vi "FGV_viertel_kreis_1Q.vi"(8 "error in (no error)":errorcluster, 9 "Sektor":T1, 11 "mode":T2) -> (0 "error out":errorcluster, 1 "size":i32, 3 "Q":dbl[][](array[numeric]) format="%_2g")   [LabVIEW 2019]
uses:
  mode_Q.ctl
  Quadrant.ctl
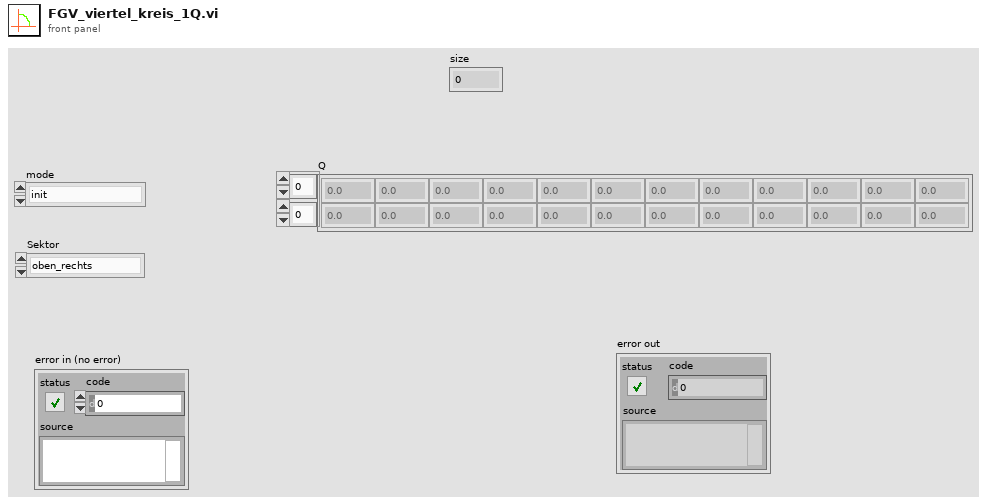
[diagram p1: front panel]
types:
  T1 = typedef "Quadrant.ctl" = enum16{"oben_rechts", "oben_links", "unten_links", "unten_rechts"}
  T2 = typedef "mode_Q.ctl" = enum16{"init", "get"}
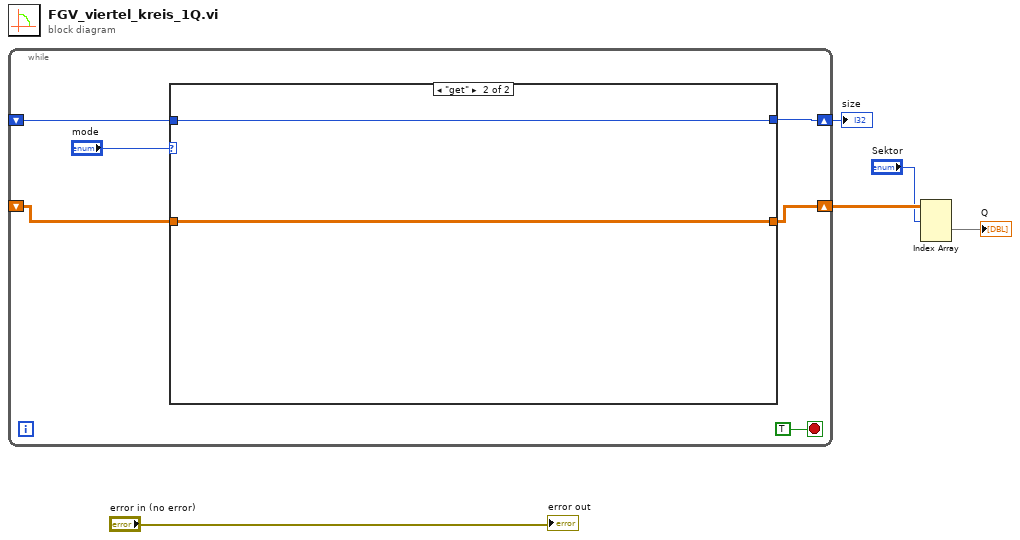
[diagram p0: block diagram]
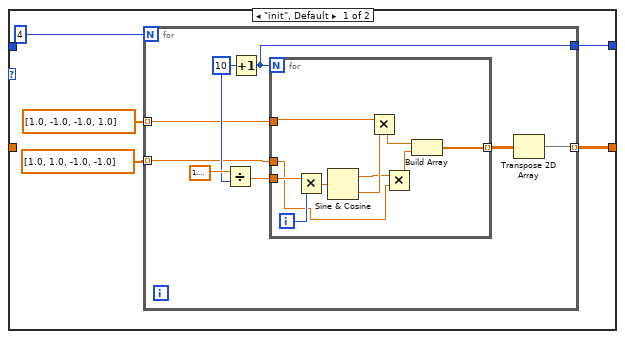
[diagram p2: hidden frame]
diagram:
  n1 = while {
    shift-right: [w9] -> w5
    shift-left: _ -> [w8]
    shift-right: [w7] -> w2
    shift-left: _ -> [w6]
    stop <- TRUE stop-if-true
    n2 = case shown="\"get\"" "mode" {
      tunnel: [w16 w36] -> w9
      tunnel: w8 -> [_ w36]
      tunnel: [w12 w35] -> w7
      tunnel: w6 -> [_ w35]
      frame "init", Default {
        n3 = for {
          N: 4 -> [_]
          tunnel: [w20] -> w16 mode=indexing
          tunnel: dbl[] [1.0, -1.0, -1.0, 1.0] -> [w19] mode=indexing
          tunnel: dbl[] [1.0, 1.0, -1.0, -1.0] -> [w18] mode=indexing
          tunnel: [w17] -> w12
          w23 = 10
          n4 = Divide(x=1.5707963267948966, y=w23) -> (x/y=w22:dbl)
          n5 = Increment(x=w23) -> (x+1=w17:i32)
          n6 = for {
            N: w17 -> [_]
            tunnel: w22 -> [w33]
            tunnel: [w29] -> w21 mode=indexing
            tunnel: w19 -> [w27]
            tunnel: w18 -> [w25]
            i -> [w34]
            n7 = Multiply(x=w33, y=w34) -> (x*y=w32:dbl)
            n8 = Sine & Cosine(0:w32) -> (1:w30:dbl, 2:w31:dbl)
            n9 = Multiply(x=w27, y=w31) -> (x*y=w28:dbl)
            n10 = Multiply(x=w30, y=w25) -> (x*y=w26:dbl)
            n11 = Build Array(w28, w26) -> (w29:dbl[])
          }
          n12 = Transpose 2D Array(2D array=w21) -> (transposed array=w20:dbl[][])
        }
      }
      frame "get" {
      }
    }
  }
  "size" <- w2
  n13 = Index Array(array=w5, index (dim 0)="Sektor") -> (element=→"Q":dbl[][])  [unwired: 2 in]
  "error out" <- "error in (no error)"
